vi "wait after each move.vi"   [LabVIEW 2020, in "core.lvlib"]
uses:
  core.lvlib
  core_wait (global variable).vi
panel:
  # "Development\ncontrols/indicators useful for development and testing, but which are not outputs of the VI"
  # "Input\nInputs to the VI"
  # "Output\nOutputs of the VI"
  # "Description\n\nBlank VI with error handling case. \n\nSummarize the use of this VI in this space."
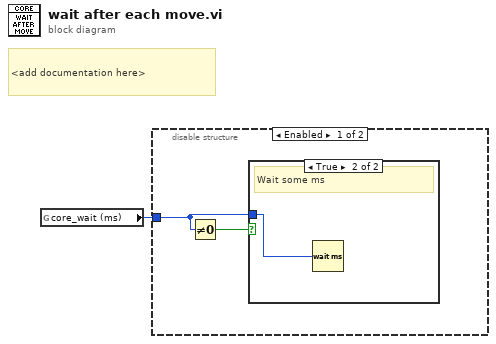
[diagram p0: block diagram]
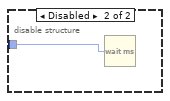
[diagram p3: hidden frame]
diagram:
  # "<add documentation here>"
  n1 = global read "core_wait (global variable).vi" "core_wait (ms)"() -> (w1:u32)
  n2 = disable-structure shown="Enabled" {
    disable-tunnel: w1 -> [w2 w5]
    frame Enabled {
      n3 = Not Equal To 0?(x=w2) -> (x != 0?=w3:bool)
      n4 = case shown="True" w3 {
        tunnel: w2 -> [_ w4]
        frame False {
          # "Wait 0 ms. Do nothing."
        }
        frame True {
          # "Wait some ms"
          n5 = Wait (ms)(milliseconds to wait=w4) -> ()  [unwired: 1 out]
        }
      }
    }
    frame Disabled {
      n6 = Wait (ms)(milliseconds to wait=w5) -> ()  [unwired: 1 out]
    }
  }
